vi "adjustAngle_04.vi"() -> ()   [LabVIEW 2011]
panel:
  in  "first":bool=TRUE
  out "tStart":dbl
  in  "Move to ref angle first":bool=TRUE
  in  "time done (s)":dbl
  in  "time to wait (s)":dbl=2.0
  out "Wait to set":bool
  in  "dAngle (deg)":dbl=30.0 format="%.1f"
  out "IO error":errorcluster
  in  "stop":bool
  out "Angle Indicator (deg)":dbl=20.6 caption="Angle (deg)" format="%.1f"
  in  "Angle (deg)":dbl format="%.1f"
  out "P (torr)":dbl=19.959999999999997 format="%.2f"
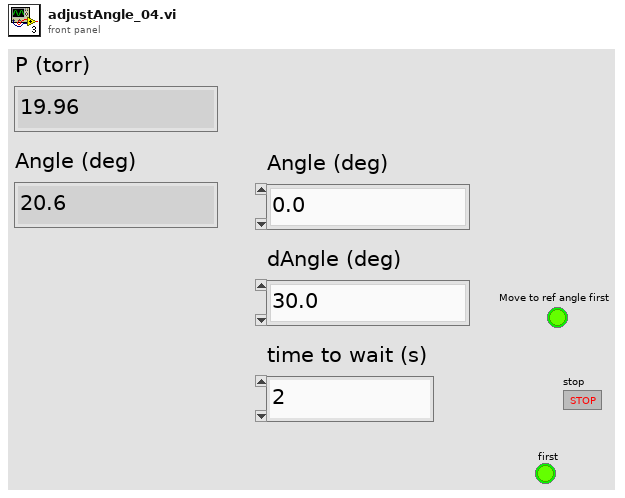
[diagram p1: front panel]
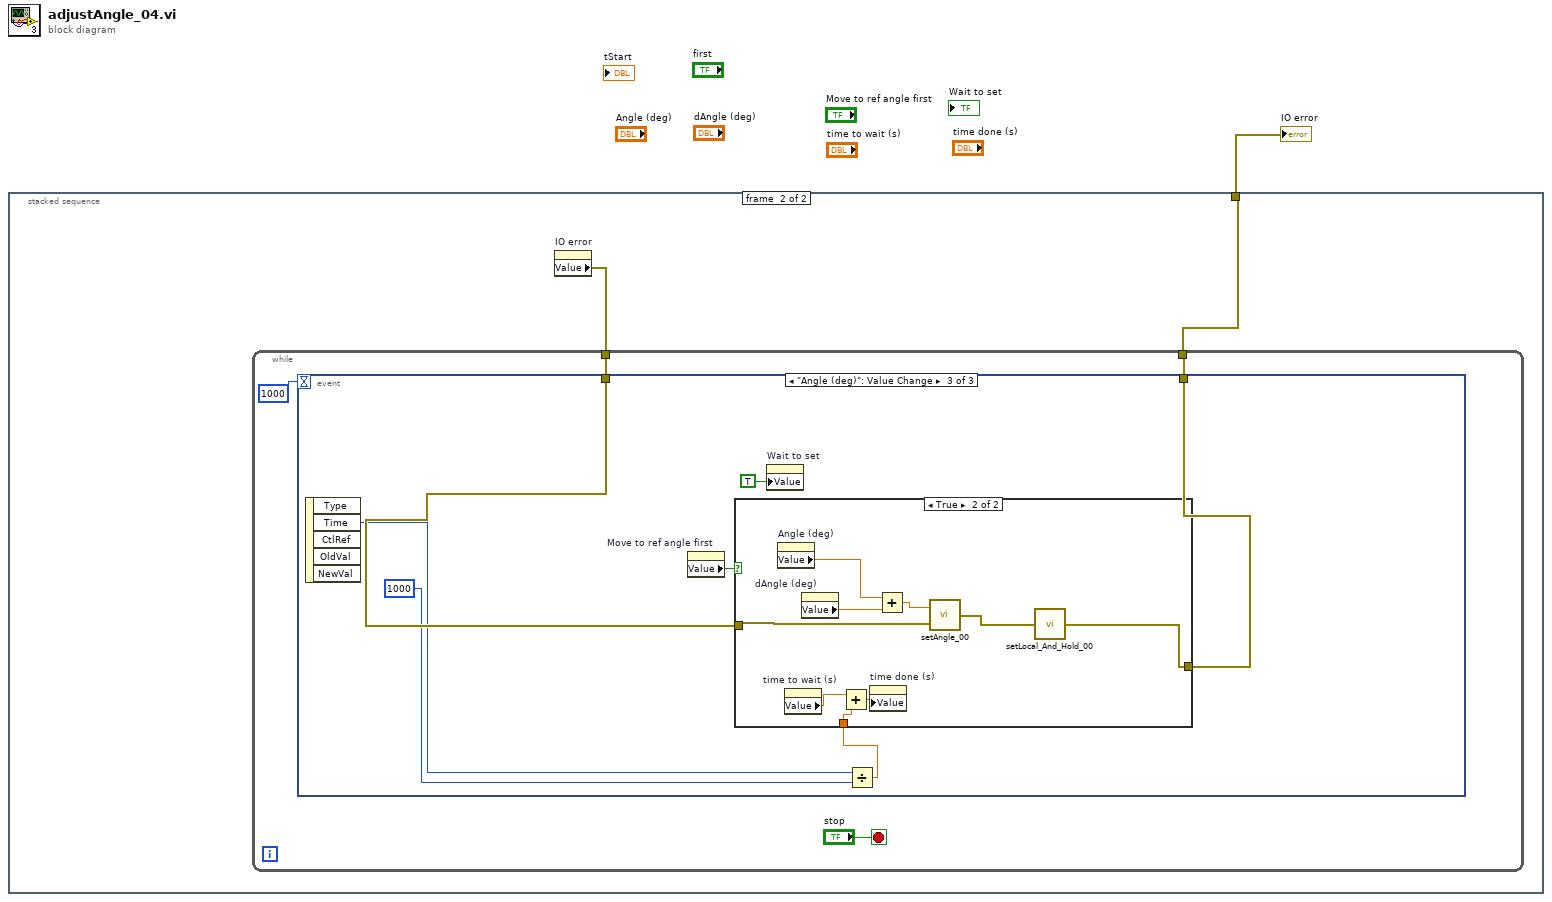
[diagram p0: block diagram]
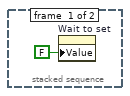
[diagram p2: hidden frame]
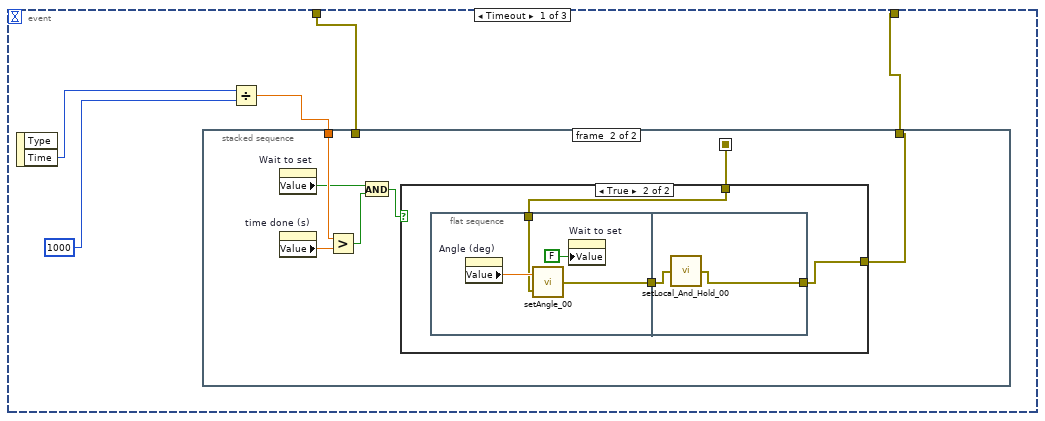
[diagram p3: hidden frame]
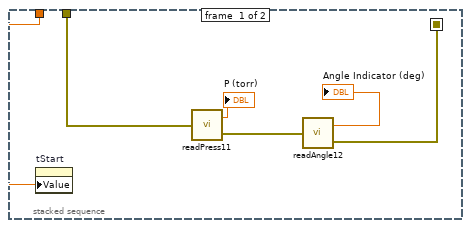
[diagram p4: hidden frame]
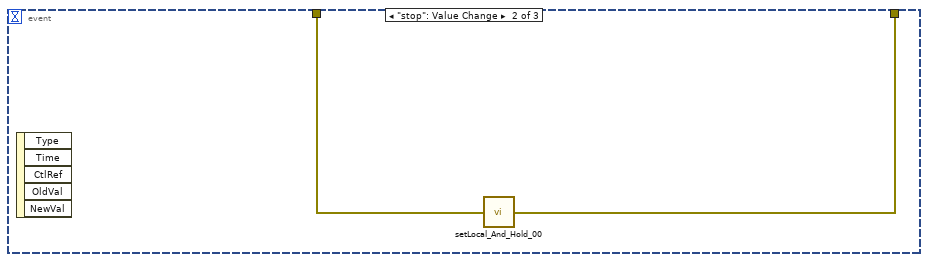
[diagram p6: hidden frame]
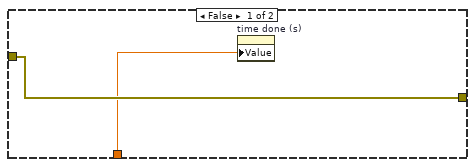
[diagram p7: hidden frame]
diagram:
  n1 = stacked-sequence {
    tunnel: [_ w3] -> w1
    frame #0 {
      n2 = property on="Wait to set" class="Bool (strict)"("Value"=FALSE ("Wait to set")) -> ()  [unwired: 2 in, 2 out]
    }
    frame #1 {
      n3 = property on="IO error" class="Clust (strict)"() -> ("Value"=w4:errorcluster)  [unwired: 2 in, 2 out]
      n4 = while {
        tunnel: w4 -> [w7]
        tunnel: [w6] -> w3
        stop <- "stop" stop-if-true
        n5 = event shown="[2] \"Angle (deg)\": Value Change" {
          selector: _ -> [_ _ _]
          dyn-events: _ -> [_ _ _]
          timeout: 1000 -> [_ _ _]
          tunnel: w7 -> [w13 w38 w44]
          tunnel: [w12 w37 w45] -> w6
          event Timeout {
            n6 = event-data() -> ("Time"=w11:u32)  [unwired: 1 in, 1 out]
            n7 = Divide(x=w11, y=u32 1000) -> (x/y=w9:dbl)
            n8 = stacked-sequence {
              seq-local: [w15 _] -> [_ w20]
              tunnel: w13 -> [w19 _]
              tunnel: w9 -> [w14 w26]
              tunnel: [_ w22] -> w12
              frame #0 {
                n9 = property on="tStart" class="DigNum (strict)"("Value"=w14) -> ()  [unwired: 2 in, 2 out]
                n10 = call "readPress11.vi"("error in"=w19) -> ("P"=→"P (torr)":dbl, "error out"=w16:errorcluster)
                n11 = call "readAngle12.vi"("error in"=w16) -> ("angle"=→"Angle Indicator (deg)":dbl, "error out"=w15:errorcluster)
              }
              frame #1 {
                n12 = property on="Wait to set" class="Bool (strict)"() -> ("Value"=w21:bool)  [unwired: 2 in, 2 out]
                n13 = property on="time done (s)" class="DigNum (strict)"() -> ("Value"=w25:dbl)  [unwired: 2 in, 2 out]
                n14 = Greater?(x=w26, y=w25) -> (0:w24:bool)
                n15 = And(x=w21, y=w24) -> (x .and. y?=w23:bool)
                n16 = case shown="True" w23 {
                  tunnel: [w27 w30] -> w22
                  tunnel: w20 -> [w27 w28]
                  frame False {
                  }
                  frame True {
                    n17 = flat-sequence {
                      tunnel: [w33] -> w29
                      tunnel: w28 -> [w31]
                      tunnel: [w35] -> w30
                      tunnel: w29 -> [w36]
                      frame #0 {
                        n18 = property on="Angle (deg)" class="DigNum (strict)"() -> ("Value"=w34:dbl)  [unwired: 2 in, 2 out]
                        n19 = call "setAngle_00.vi"("error in (no error)"=w31, "Angle (deg)"=w34) -> ("error out"=w33:errorcluster)
                        n20 = property on="Wait to set" class="Bool (strict)"("Value"=FALSE ("Wait to set")) -> ()  [unwired: 2 in, 2 out]
                      }
                      frame #1 {
                        n21 = call "setLocal_And_Hold_00.vi"("error in (no error)"=w36) -> ("error out"=w35:errorcluster)
                      }
                    }
                  }
                }
              }
            }
          }
          event "stop": Value Change {
            n22 = event-data() -> ()  [unwired: 1 in, 5 out]
            n23 = call "setLocal_And_Hold_00.vi"("error in (no error)"=w38) -> ("error out"=w37:errorcluster)
          }
          event "Angle (deg)": Value Change {
            n24 = event-data() -> ("Time"=w43:u32)  [unwired: 1 in, 4 out]
            n25 = property on="Move to ref angle first" class="Bool (strict)"() -> ("Value"=w40:bool)  [unwired: 2 in, 2 out]
            n26 = property on="Wait to set" class="Bool (strict)"("Value"=TRUE ("Wait to set")) -> ()  [unwired: 2 in, 2 out]
            n27 = Divide(x=w43, y=u32 1000) -> (x/y=w41:dbl)
            n28 = case shown="True" w40 {
              tunnel: w44 -> [w47 w56]
              tunnel: [w47 w51] -> w45
              tunnel: w41 -> [w46 w53]
              frame False {
                n29 = property on="time done (s)" class="DigNum (strict)"("Value"=w46) -> ()  [unwired: 2 in, 2 out]
              }
              frame True {
                n30 = property on="Angle (deg)" class="DigNum (strict)"() -> ("Value"=w49:dbl)  [unwired: 2 in, 2 out]
                n31 = property on="time to wait (s)" class="DigNum (strict)"() -> ("Value"=w54:dbl)  [unwired: 2 in, 2 out]
                n32 = property on="dAngle (deg)" class="DigNum (strict)"() -> ("Value"=w50:dbl)  [unwired: 2 in, 2 out]
                n33 = Add(x=w54, y=w53) -> (x+y=w55:dbl)
                n34 = property on="time done (s)" class="DigNum (strict)"("Value"=w55) -> ()  [unwired: 2 in, 2 out]
                n35 = Add(x=w49, y=w50) -> (x+y=w48:dbl)
                n36 = call "setAngle_00.vi"("error in (no error)"=w56, "Angle (deg)"=w48) -> ("error out"=w52:errorcluster)
                n37 = call "setLocal_And_Hold_00.vi"("error in (no error)"=w52) -> ("error out"=w51:errorcluster)
              }
            }
          }
        }
      }
    }
  }
  "IO error" <- w1
